vi "Filter_SubVI.vi"(8 "Enable":bool, 9 "Highpass Freq":dbl, 10 "sample rate (S/s)":dbl, 11 "Signal Array":dbl[](array[numeric])) -> (3 "Filtered X":dbl[](array[numeric]))   [LabVIEW 2024]
doc: "This SubVI takes the sample rate and highpass Freq and uses it to add a lowpass filter onto a signal.\n\nIN: Signal Array, Sample Rate; Highpass Freq; Enable;\nOUT: Filtered Signal Array;"
uses:
  <vilib>/Analysis/3filter.llb/Filter Passband Type.ctl
  <vilib>/Analysis/3filter.llb/Bessel Filter (DBL).vi
  <vilib>/Analysis/NI_AALBase.lvlib
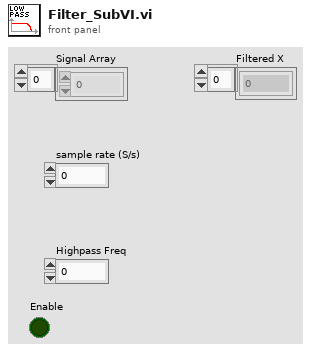
[diagram p1: front panel]
types:
  T1 = typedef "NI_AALBase.lvlib/Filter Passband Type.ctl" = enum32{"Lowpass", "Highpass", "Bandpass", "Bandstop"}
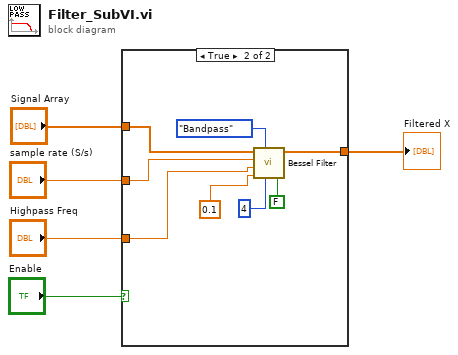
[diagram p0: block diagram]
diagram:
  n1 = case shown="True" "Enable" {
    tunnel: "Highpass Freq" -> [_ w8]
    tunnel: "sample rate (S/s)" -> [_ w12]
    tunnel: [w6 w9] -> w3
    tunnel: "Signal Array" -> [w6 w11]
    frame False {
    }
    frame True {
      n2 = call-poly <vilib>:"Bessel Filter.vi"("init/cont (init:F)"=FALSE, "order"=4, "filter type"=Filter_Passband_Type."Bandpass", "low cutoff freq: fl"=0.1, "high cutoff freq: fh"=w8, "sampling freq: fs"=w12, "X"=w11) -> ("Filtered X"=w9:dbl[])  [unwired: 1 in, 1 out]
    }
  }
  "Filtered X" <- w3
